vi "Configure Device.vi"(8 "error in":errorcluster, 11 "Meerstetter TEC in":refnum<class "Meerstetter TEC.lvclass">) -> (0 "error out":errorcluster, 2 "CfgDataOut":string, 3 "Meerstetter TEC out":refnum<class "Meerstetter TEC.lvclass">, 4 "SP":dbl, 5 "Settable?":bool)   [LabVIEW 2014, in "Meerstetter Lib.lvlib" / "Meerstetter TEC.lvclass"]
uses:
  Meerstetter TEC.lvclass
  reusable/Session APIs/Serial/Serial Session.lvclass
  Configurable Device/Configurable Device.lvclass/Configurable Device.ctl
  Meerstetter TEC.lvclass/Meerstetter TEC.ctl
  Controls/Ctl Method.ctl
  reusable/Session APIs/File Access/Config Data/Config Data.lvclass/Config Data.ctl
  Controls/Input Selection.ctl
  Configurable Device/Read ID.vi
  reusable/Session APIs/File Access/Config Data/Accessors/Read Ref.vi
  Accessors/Write ctlVal.vi
  Accessors/Write Address.vi
  Configurable Device/Read Handle.vi
  Accessors/Write SerialSession.vi
  <vilib>/Utility/config.llb/Read Key (String).vi
  <vilib>/Utility/config.llb/Read Key (U32).vi
  <vilib>/Utility/config.llb/Read Key (Double).vi
  reusable/Session APIs/File Access/Config Data/Config Data.lvclass
  <vilib>/Utility/config.llb/NI_LVConfig.lvlib
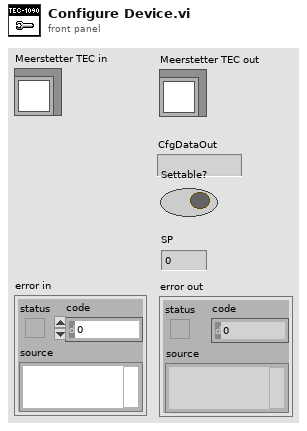
[diagram p1: front panel]
types:
  T1 = typedef "Serial Session.lvclass/Session Handle.ctl" = refnum<data-value>
  T2 = typedef "Config Data.lvclass/Config Session.ctl" = refnum<data-value>
  T3 = typedef "Ctl Method.ctl" = enum16{"Temperature", "Power"}
  T4 = typedef "Input Selection.ctl" = enum16{"Static Current/Voltage", "Live Current/Voltage", "Temperature Controller"}
  T5 = typedef "NI_LVConfig.lvlib/Config Data RefNum.ctl" = refnum<k1>
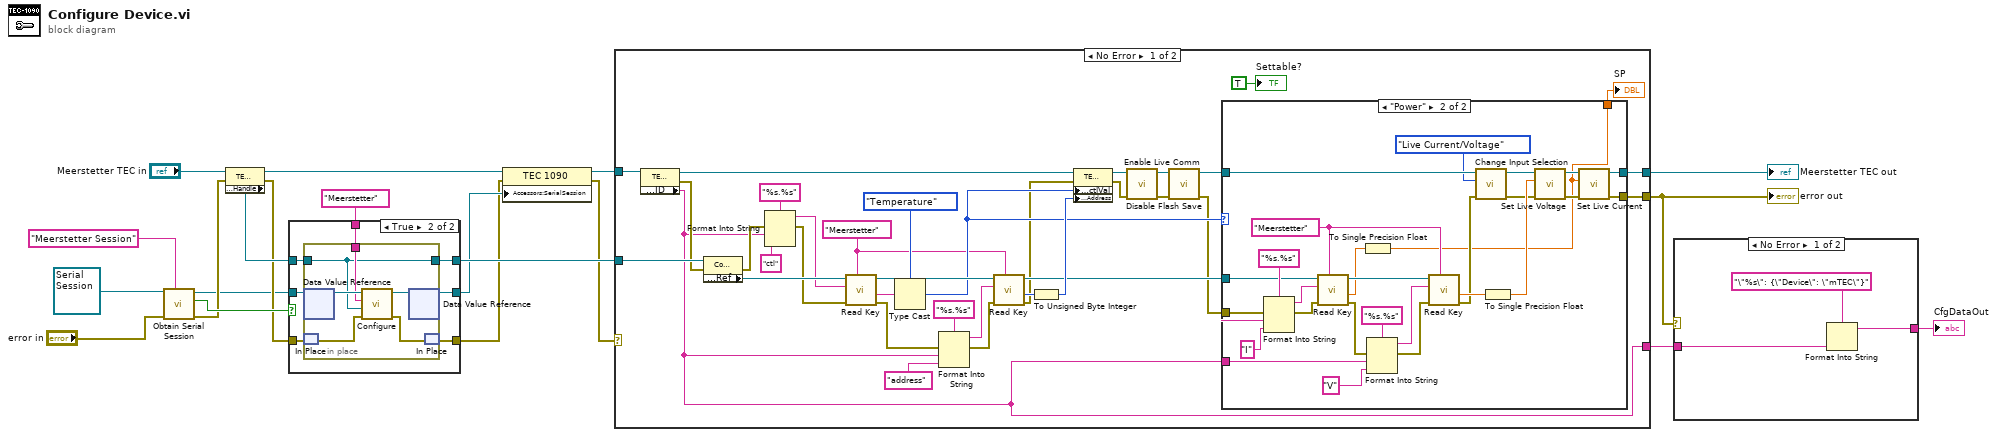
[diagram p0: block diagram]
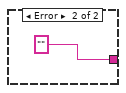
[diagram p2: hidden frame]
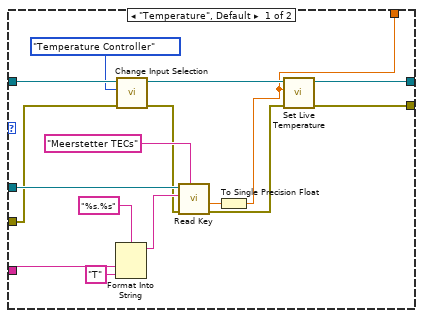
[diagram p3: hidden frame]
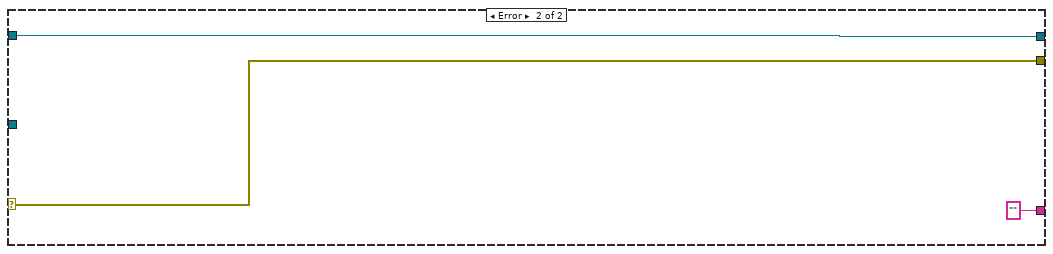
[diagram p4: hidden frame]
diagram:
  n1 = call "Obtain Serial Session.vi"("Session Name ()"="Meerstetter Session", "error in"="error in", "Serial Session in"=refnum<class "Serial Session.lvclass"> refnum) -> ("error out"=w17:errorcluster, "created new?"=w20:bool, "hSerial"=w15:T1)  [unwired: 6 in]
  n2 = property class="TEC 1090"(reference="Meerstetter TEC in", error in=w17) -> (reference out=w8:refnum<class "Meerstetter TEC.lvclass">, error out=w16:errorcluster, "Accessors:Handle"=w18:T2)
  n3 = case shown="True" w20 {
    tunnel: w15 -> [w23 w30]
    tunnel: w16 -> [w22 w26]
    tunnel: [w23 w29] -> w6
    tunnel: [w22 w28] -> w4
    tunnel: w18 -> [w21 w27]
    tunnel: [w21 w25] -> w11
    tunnel: "Meerstetter" ("section") -> [_ w24]
    frame False {
    }
    frame True {
      n4 = in-place {
        in-place-border: w27 -> [w31]
        in-place-border: w24 -> [w32]
        in-place-border: [w31] -> w25
        n5 = in-place-dvr #1(w30) -> (w36:refnum<class "Serial Session.lvclass">)  [unwired: 1 out]
        n6 = in-place-match #2(w26) -> (w35:errorcluster)
        n7 = call "Configure.vi"("error in"=w35, "Config Handle"=w31, "section"=w32, "Serial Session in"=w36) -> ("error out"=w34:errorcluster, "Serial Session out"=w33:refnum<class "Serial Session.lvclass">)  [unwired: 6 in]
        n8 = in-place-dvr #1(w33) -> (w29:T1)  [unwired: 1 out]
        n9 = in-place-match #2(w34) -> (w28:errorcluster)
      }
    }
  }
  n10 = property class="TEC 1090"(reference=w8, error in=w4, "Accessors:SerialSession"=w6) -> (reference out=w7:refnum<class "Meerstetter TEC.lvclass">, error out=w5:errorcluster)
  n11 = case shown="No Error" w5 {
    selector: w5 -> [_ w116]
    tunnel: w7 -> [w69 w117]
    tunnel: w11 -> [w71 _]
    tunnel: [w51 w117] -> w10
    tunnel: [w50 w116] -> w3
    tunnel: [w39 "" ("Accessors:ID")] -> w1
    frame No Error {
      w49 = "Meerstetter" ("section")
      n12 = property class="TEC 1090"(reference=w69) -> (reference out=w63:refnum<class "Meerstetter TEC.lvclass">, error out=w48:errorcluster, "Accessors:ID"=w39:string)  [unwired: 1 in]
      n13 = property class="Config Data"(reference=w71, error in=w48) -> (error out=w47:errorcluster, "Accessors:Ref"=w70:T5)  [unwired: 1 out]
      n14 = Format Into String(format string="%s.%s", error in=w47, w39, "ctl" ("input 2")) -> (resulting string=w66:string, error out=w46:errorcluster)  [unwired: 1 in]
      n15 = call-poly <vilib>:"Read Key.vi"("section"=w49, "error in (no error)"=w46, "key"=w66, "refnum"=w70) -> ("error out"=w45:errorcluster, "value"=w65:string, "refnum out"=w62:T5)  [unwired: 4 in, 1 out]
      n16 = Type Cast(type=Ctl_Method."Temperature" ("ctlVal"), x=w65) -> (*(type *) &x=w56:T3)
      n17 = Format Into String(format string="%s.%s", error in=w45, w39, "address" ("input 2")) -> (resulting string=w59:string, error out=w44:errorcluster)  [unwired: 1 in]
      n18 = call-poly <vilib>:"Read Key.vi"("section"=w49, "error in (no error)"=w44, "key"=w59, "refnum"=w62) -> ("error out"=w54:errorcluster, "value"=w58:u32, "refnum out"=w55:T5)  [unwired: 4 in, 1 out]
      n19 = To Unsigned Byte Integer(number=w58) -> (unsigned 8bit integer=w57:u8)
      n20 = property class="TEC 1090"(reference=w63, error in=w54, "Accessors:ctlVal"=w56, "Accessors:Address"=w57) -> (reference out=w53:refnum<class "Meerstetter TEC.lvclass">, error out=w43:errorcluster)
      n21 = call "Disable Flash Save.vi"("error in"=w43, "TEC 1090 in"=w53) -> ("error out"=w40:errorcluster, "TEC 1090 out"=w41:refnum<class "Meerstetter TEC.lvclass">)  [unwired: 8 in]
      n22 = call "Enable Live Comm.vi"("error in"=w40, "TEC 1090 in"=w41) -> ("error out"=w42:errorcluster, "TEC 1090 out"=w52:refnum<class "Meerstetter TEC.lvclass">)  [unwired: 8 in]
      n23 = case shown="\"Power\"" w56 {
        tunnel: w39 -> [w82 w110]
        tunnel: w55 -> [w84 w108]
        tunnel: w52 -> [w81 w99]
        tunnel: [w76 w100] -> w51
        tunnel: [w75 w93] -> w50
        tunnel: w42 -> [w73 w92]
        tunnel: [w72 w88] -> w38
        frame "Temperature", Default {
          n24 = Format Into String(format string="%s.%s", w82, "T" ("input 2")) -> (resulting string=w85:string)  [unwired: 2 in, 1 out]
          n25 = call "Change Input Selection.vi"("error in"=w73, "Input Selection"=Input_Selection."Temperature Controller", "TEC 1090 in"=w81) -> ("error out"=w79:errorcluster, "TEC 1090 out"=w77:refnum<class "Meerstetter TEC.lvclass">)  [unwired: 7 in]
          n26 = call-poly <vilib>:"Read Key.vi"("section"="Meerstetter TECs", "error in (no error)"=w79, "key"=w85, "refnum"=w84) -> ("error out"=w74:errorcluster, "value"=w78:dbl)  [unwired: 4 in, 2 out]
          n27 = To Single Precision Float(number=w78) -> (single precision float=w72:sgl)
          n28 = call "Set Live Temperature.vi"("error in"=w74, "T"=w72, "TEC 1090 in"=w77) -> ("error out"=w75:errorcluster, "TEC 1090 out"=w76:refnum<class "Meerstetter TEC.lvclass">)  [unwired: 7 in]
        }
        frame "Power" {
          w105 = "Meerstetter" ("section")
          n29 = Format Into String(format string="%s.%s", error in=w92, w110, "I" ("input 2")) -> (resulting string=w109:string, error out=w91:errorcluster)  [unwired: 1 in]
          n30 = call-poly <vilib>:"Read Key.vi"("section"=w105, "error in (no error)"=w91, "key"=w109, "refnum"=w108) -> ("error out"=w90:errorcluster, "value"=w103:dbl, "refnum out"=w107:T5)  [unwired: 4 in, 1 out]
          n31 = To Single Precision Float(number=w103) -> (single precision float=w88:sgl)
          n32 = Format Into String(format string="%s.%s", error in=w90, w110, "V" ("input 2")) -> (resulting string=w106:string, error out=w89:errorcluster)  [unwired: 1 in]
          n33 = call-poly <vilib>:"Read Key.vi"("section"=w105, "error in (no error)"=w89, "key"=w106, "refnum"=w107) -> ("error out"=w96:errorcluster, "value"=w104:dbl)  [unwired: 4 in, 2 out]
          n34 = call "Change Input Selection.vi"("error in"=w96, "Input Selection"=Input_Selection."Live Current/Voltage", "TEC 1090 in"=w99) -> ("error out"=w95:errorcluster, "TEC 1090 out"=w98:refnum<class "Meerstetter TEC.lvclass">)  [unwired: 7 in]
          n35 = To Single Precision Float(number=w104) -> (single precision float=w102:sgl)
          n36 = call "Set Live Voltage.vi"("error in"=w95, "V"=w102, "TEC 1090 in"=w98) -> ("error out"=w94:errorcluster, "TEC 1090 out"=w101:refnum<class "Meerstetter TEC.lvclass">)  [unwired: 7 in]
          n37 = call "Set Live Current.vi"("error in"=w94, "I"=w88, "TEC 1090 in"=w101) -> ("error out"=w93:errorcluster, "TEC 1090 out"=w100:refnum<class "Meerstetter TEC.lvclass">)  [unwired: 7 in]
        }
      }
      "SP" <- w38
      "Settable?" <- TRUE ("Settable?")
    }
    frame Error {
    }
  }
  "error out" <- w3
  "Meerstetter TEC out" <- w10
  n38 = case shown="No Error" w3 {
    tunnel: [w119 ""] -> w2
    tunnel: w1 -> [w118 _]
    frame No Error {
      n39 = Format Into String(format string="\"%s\": {\"Device\": \"mTEC\"}", w118) -> (resulting string=w119:string)  [unwired: 2 in, 1 out]
    }
    frame Error {
    }
  }
  "CfgDataOut" <- w2
